vi "Eth Status Read Write Enables.vi"(7 "Status Reference":T1, 8 "error in (no error)":errorcluster, 10 "Lenght":i32, 11 "Index":i32) -> (0 "error out":errorcluster, 2 "WrEn":bool[](array[boolean]))   [LabVIEW 2021, in "Eth Status.lvlib"]
uses:
  Eth Status.lvlib
  Ctl/Status.ctl
  MB_TCP2/MB_TCP_State.ctl
  MB_TCP2/MB_TCP.lvclass
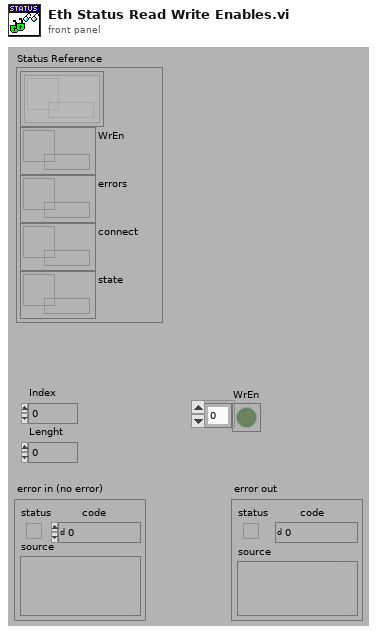
[diagram p1: front panel]
types:
  T1 = typedef "Eth Status.lvlib/Status.ctl" = cluster{"Set_states":refnum<queue>[], "WrEn":refnum<data-value>, "errors":refnum<data-value>, "connect":refnum<data-value>, "state":refnum<data-value>}
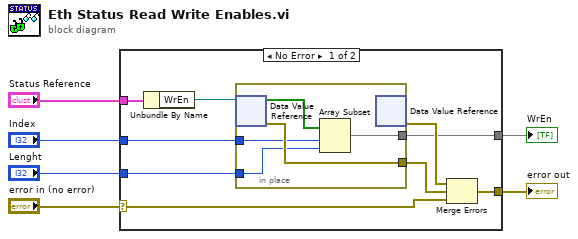
[diagram p0: block diagram]
diagram:
  n1 = case shown="No Error" "error in (no error)" {
    selector: "error in (no error)" -> [w7 w21]
    tunnel: [w13 w21] -> w6
    tunnel: "Index" -> [w15 _]
    tunnel: "Status Reference" -> [w14 _]
    tunnel: "Lenght" -> [w10 _]
    tunnel: [w8 _] -> w2
    frame No Error {
      n2 = Unbundle By Name(w14) -> ("WrEn"=w11:refnum<data-value>)
      n3 = in-place {
        in-place-border: w15 -> [w18]
        in-place-border: [w20] -> w9
        in-place-border: w10 -> [w17]
        in-place-border: [w16] -> w8
        n4 = in-place-dvr #1(w11) -> (w19:bool[], w20:errorcluster)
        n5 = Array Subset(array=w19, index=w18, length=w17) -> (w16:bool[])
        n6 = in-place-dvr #1() -> (w12:errorcluster)  [unwired: 1 in, 1 out]
      }
      n7 = Merge Errors(w12, w9, w7) -> (w13:errorcluster)
    }
    frame Error {
    }
  }
  "error out" <- w6
  "WrEn" <- w2
